vi "Report Diagnostics.vi"(8 "error in (no error)":errorcluster, 9 "Finished Late? [i-1]":bool, 10 "Iteration Duration":i64, 11 "Data Value Reference in":T1) -> (0 "error out":errorcluster)   [LabVIEW 2017, in "NI 272x Resistive Simulation Custom Device Engine.lvlib"]
uses:
  NI 272x Resistive Simulation Custom Device Engine.lvlib
  <vilib>/NI/NIVS Inline Async API/_Data Access Engine/Data Access Engine/Types/Write.DVR.ctl
  <vilib>/NI/NIVS Inline Async API/_Data Access Engine/Access Type Classes/Write/Write.lvclass
  <vilib>/NI/NIVS Inline Async API/_Data Access Engine/Access Type Classes/Write/Write.lvclass/Write.ctl
  <vilib>/NI/NIVS Inline Async API/_Data Access Engine/Data Access Engine/Methods/Write.Data.vi
  <vilib>/NI/NIVS Inline Async API/_Data Access Engine/Access Type Classes/Write/Write.ProcessData.vi
  <vilib>/NI/NIVS Inline Async API/_Data Access Engine/Data Access Engine/Data Access Engine.lvclass
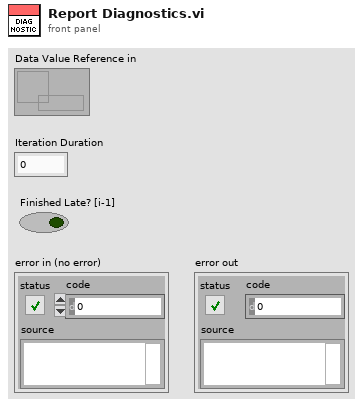
[diagram p1: front panel]
types:
  T1 = typedef "Data Access Engine.lvlib/Data Access Engine.lvclass/Write.DVR.ctl" = refnum<data-value>
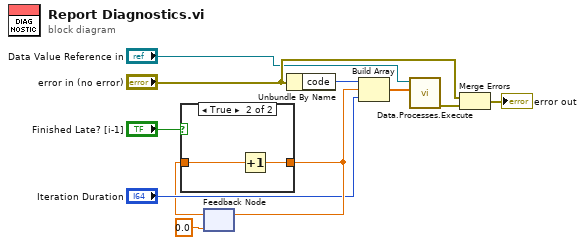
[diagram p0: block diagram]
diagram:
  n1 = feedback #1(0.0) -> (w5:dbl)
  n2 = case shown="True" "Finished Late? [i-1]" {
    tunnel: w5 -> [w12 w14]
    tunnel: [w12 w13] -> w11
    frame False {
    }
    frame True {
      n3 = Increment(x=w14) -> (x+1=w13:dbl)
    }
  }
  n4 = feedback-in #1(w11) -> ()
  n5 = Unbundle By Name("error in (no error)") -> ("code"=w3:i32)
  n6 = Build Array(w3, w11, "Iteration Duration") -> (w8:dbl[])
  n7 = call-poly <vilib>:"Data.Processes.Execute.vi"("Values"=w8, "Ref"="Data Value Reference in") -> ("error out"=w10:errorcluster)  [unwired: 9 in]
  n8 = Merge Errors("error in (no error)", w10) -> (→"error out":errorcluster)
